vi "A_PID 15_MaxRR.vi"() -> ()   [LabVIEW 2011]
uses:
  <vilib>/DAQmx/read.llb/DAQmx Read (Analog 1D DBL 1Chan NSamp).vi
  <vilib>/DAQmx/write.llb/DAQmx Write (Analog DBL 1Chan 1Samp).vi
  <vilib>/DAQmx/create/channels.llb/DAQmx Create Channel (AI-Voltage-Basic).vi
  <vilib>/DAQmx/configure/timing.llb/DAQmx Timing (Sample Clock).vi
  <vilib>/DAQmx/create/channels.llb/DAQmx Create Channel (AO-Voltage-Basic).vi
  <vilib>/DAQmx/miscellaneous.llb/DAQmx Fill In Error Info.vi
  <vilib>/express/express arith-compare/Formula/XNode/ExpressFormulaBlockNode.xnode
  <vilib>/Analysis/NI_AALBase.lvlib
  Program Files (x86)/National Instruments/LabVIEW 2011/resource/objmgr/daqmx.rc
panel:
  in  "A2":dbl=97.0
  in  "A1":dbl=98.0
  in  "error in":cluster{"status":bool}
  in  "?":T1(tab)
  in  "Go":bool
  out "Time":dbl
  out "Thermistor Back":dbl
  out "Thermistor Block":dbl
  out "Vial Ramp rate":dbl format="%#_3g"
  in  "stop":bool
  out "XY Graph":cluster{"Y":dbl[], "Y":dbl[]}[](graph)
  out "Setpoint":dbl
  in  "Zero":dbl=-0.6
  in  "Pole":dbl=-10000000000000.0
  in  "PID Heating":T2={"proportional gain (Kc)"=27.0, "integral time (Ti, s)"=8.1, "derivative time (Td, s)"=0.0} {"derivative time (Td, s)" format="%.3f"; "integral time (Ti, s)" format="%.3f"; "proportional gain (Kc)" format="%.3f"}
  out "Set Pt RampRate":dbl
  out "Error":dbl
  in  "PID Cooling":T2={"proportional gain (Kc)"=33.0, "integral time (Ti, s)"=7.0, "derivative time (Td, s)"=0.0} {"derivative time (Td, s)" format="%.3f"; "integral time (Ti, s)" format="%.3f"; "proportional gain (Kc)" format="%.3f"}
  out "Controller output":cluster{"Time Out":dbl[], dbl[]}(graph)
  out "Power Circuit":cluster{"Time Out":dbl[], dbl[]}(graph)
  out "Voltage":dbl
  out "Ave RR Up":dbl
  out "Ave RR Down":dbl
  in  "Voltage Manual":dbl=5.0
  out "volt":dbl
  in  "A3":dbl=52.0
  in  "A4":dbl=55.0
  in  "T1":dbl=16.0
  in  "T2":dbl=2.0
  in  "T3":dbl=6.0
  in  "T4":dbl=6.0
  in  "T5":dbl=12.0
  in  "T6":dbl=6.0
  in  "T7":dbl=6.0
  in  "T8":dbl=6.0
  in  "T10":dbl=6.0
  in  "T9":dbl=6.0
  in  "A6":dbl=55.0
  in  "A5":dbl=52.0
  in  "Graph Range":dbl=150.0
  out "Rate":dbl
  in  "Period(ms)":dbl=20.0
  out "time":dbl
  # "PID"
  # "Lead-Lag Compensator"
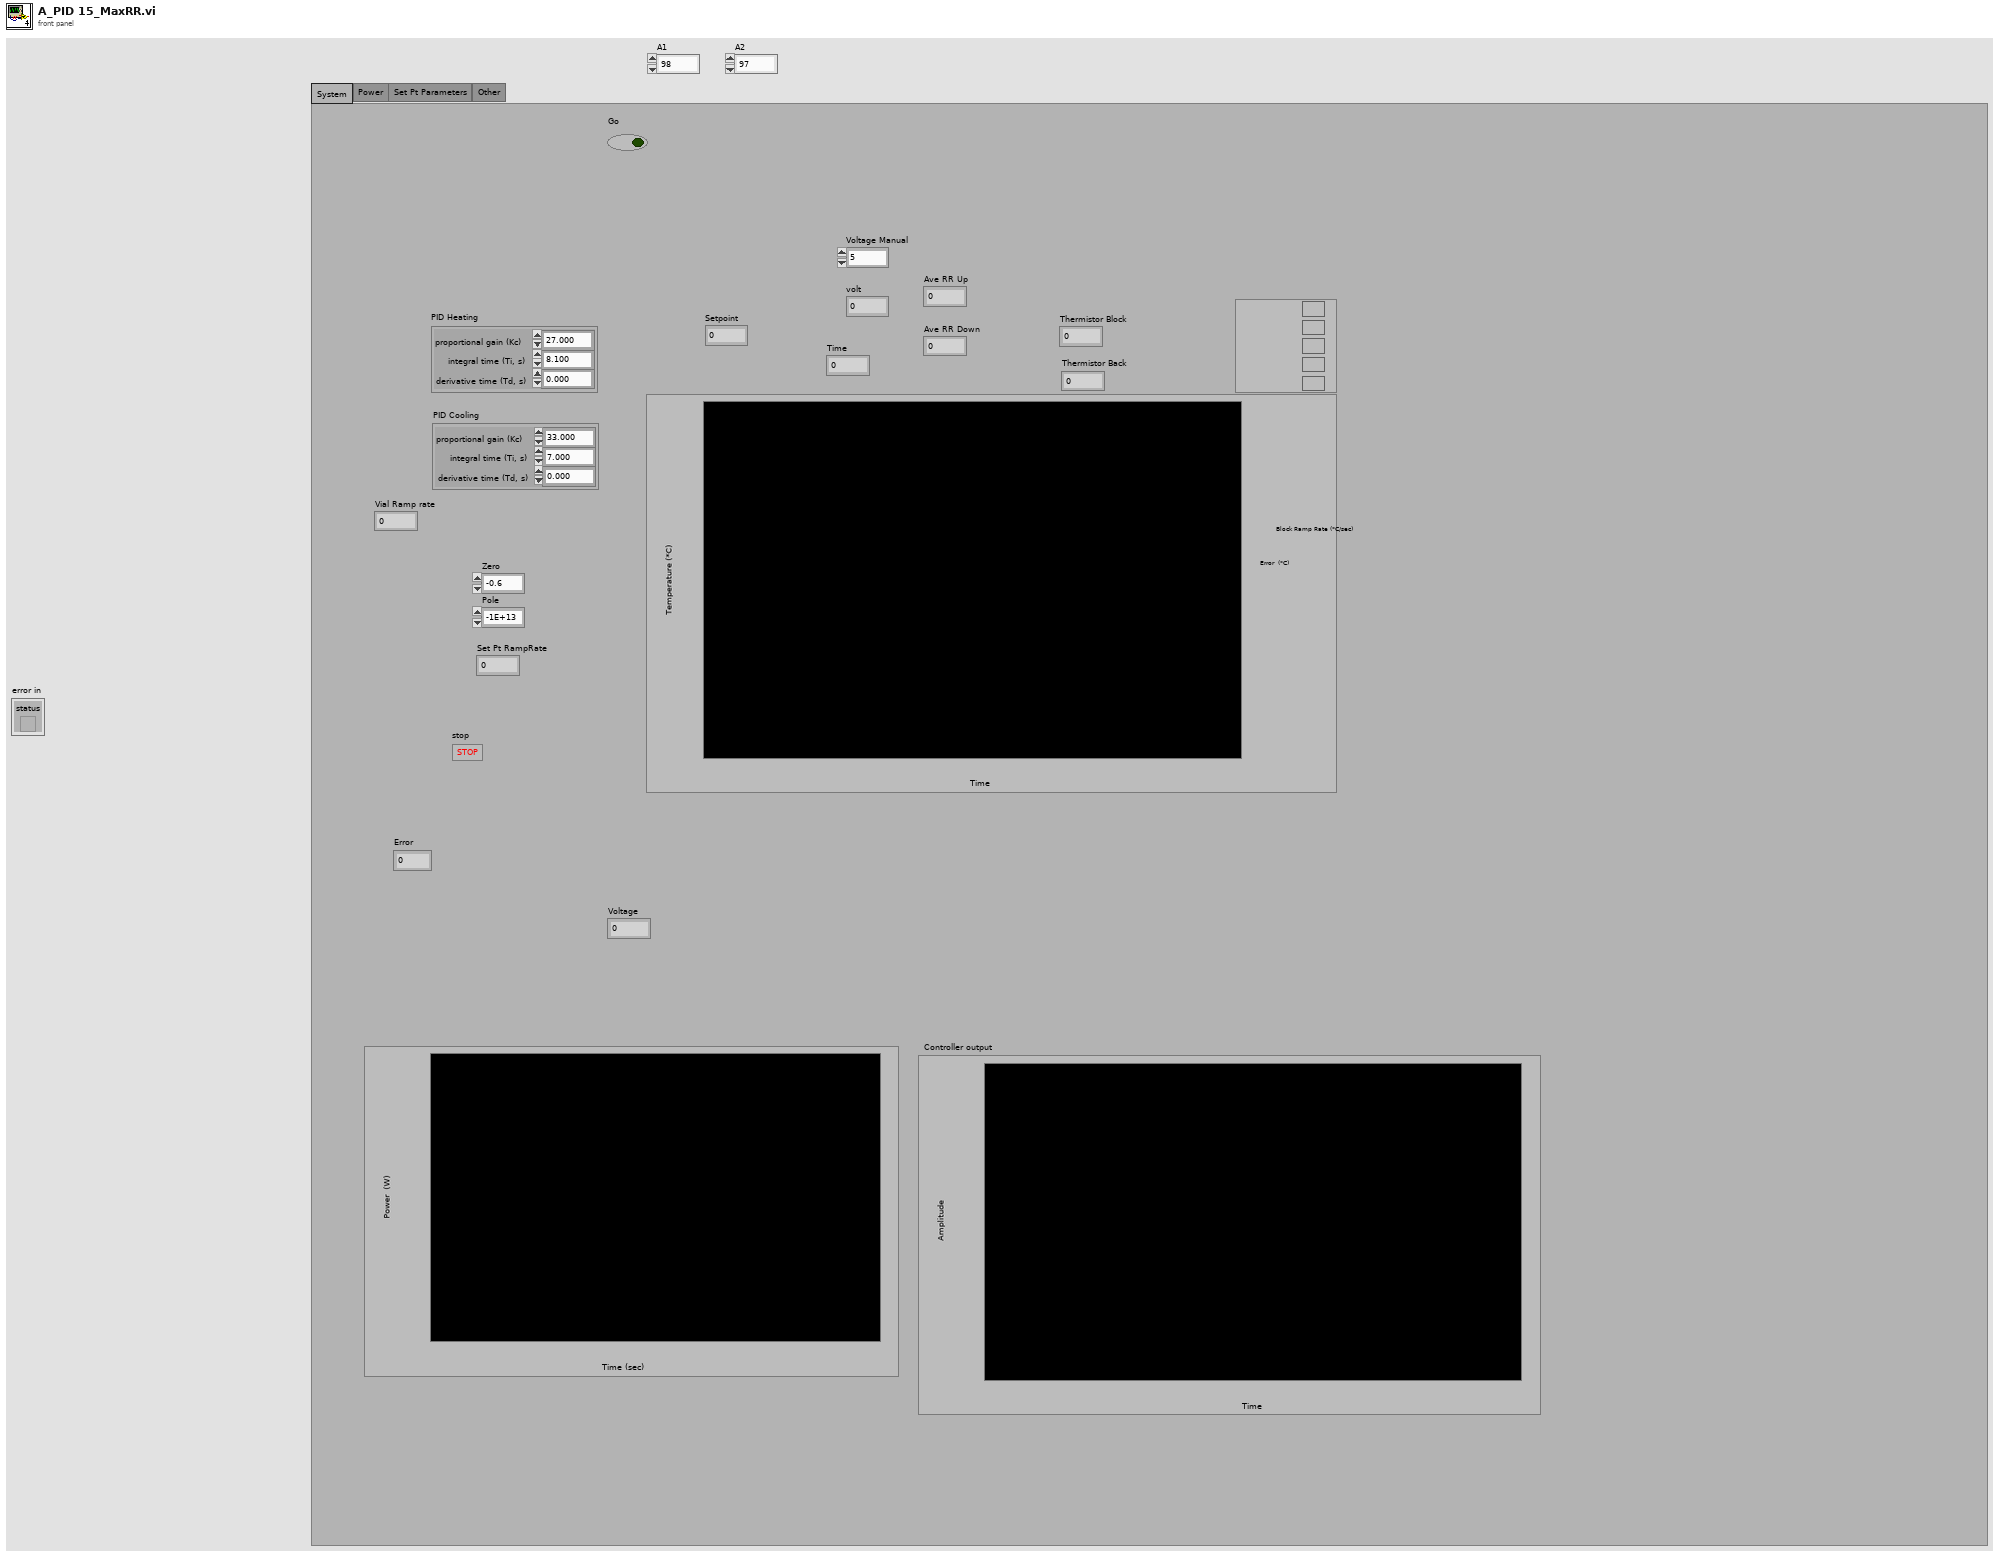
[diagram p1: front panel]
types:
  T1 = enum32{"System", "Power", "Set Pt Parameters", "Other"}
  T2 = cluster{"proportional gain (Kc)":dbl, "integral time (Ti, s)":dbl, "derivative time (Td, s)":dbl}
  T3 = enum16{"open", "replace", "create", "open or create", "replace or create", "replace or create with confirmation"}
  T4 = cluster{"x":dbl, "T1":dbl, "T2":dbl, "T3":dbl, "T4":dbl, "Te1":dbl, "Te2":dbl, "Te3":dbl, "Te4":dbl}
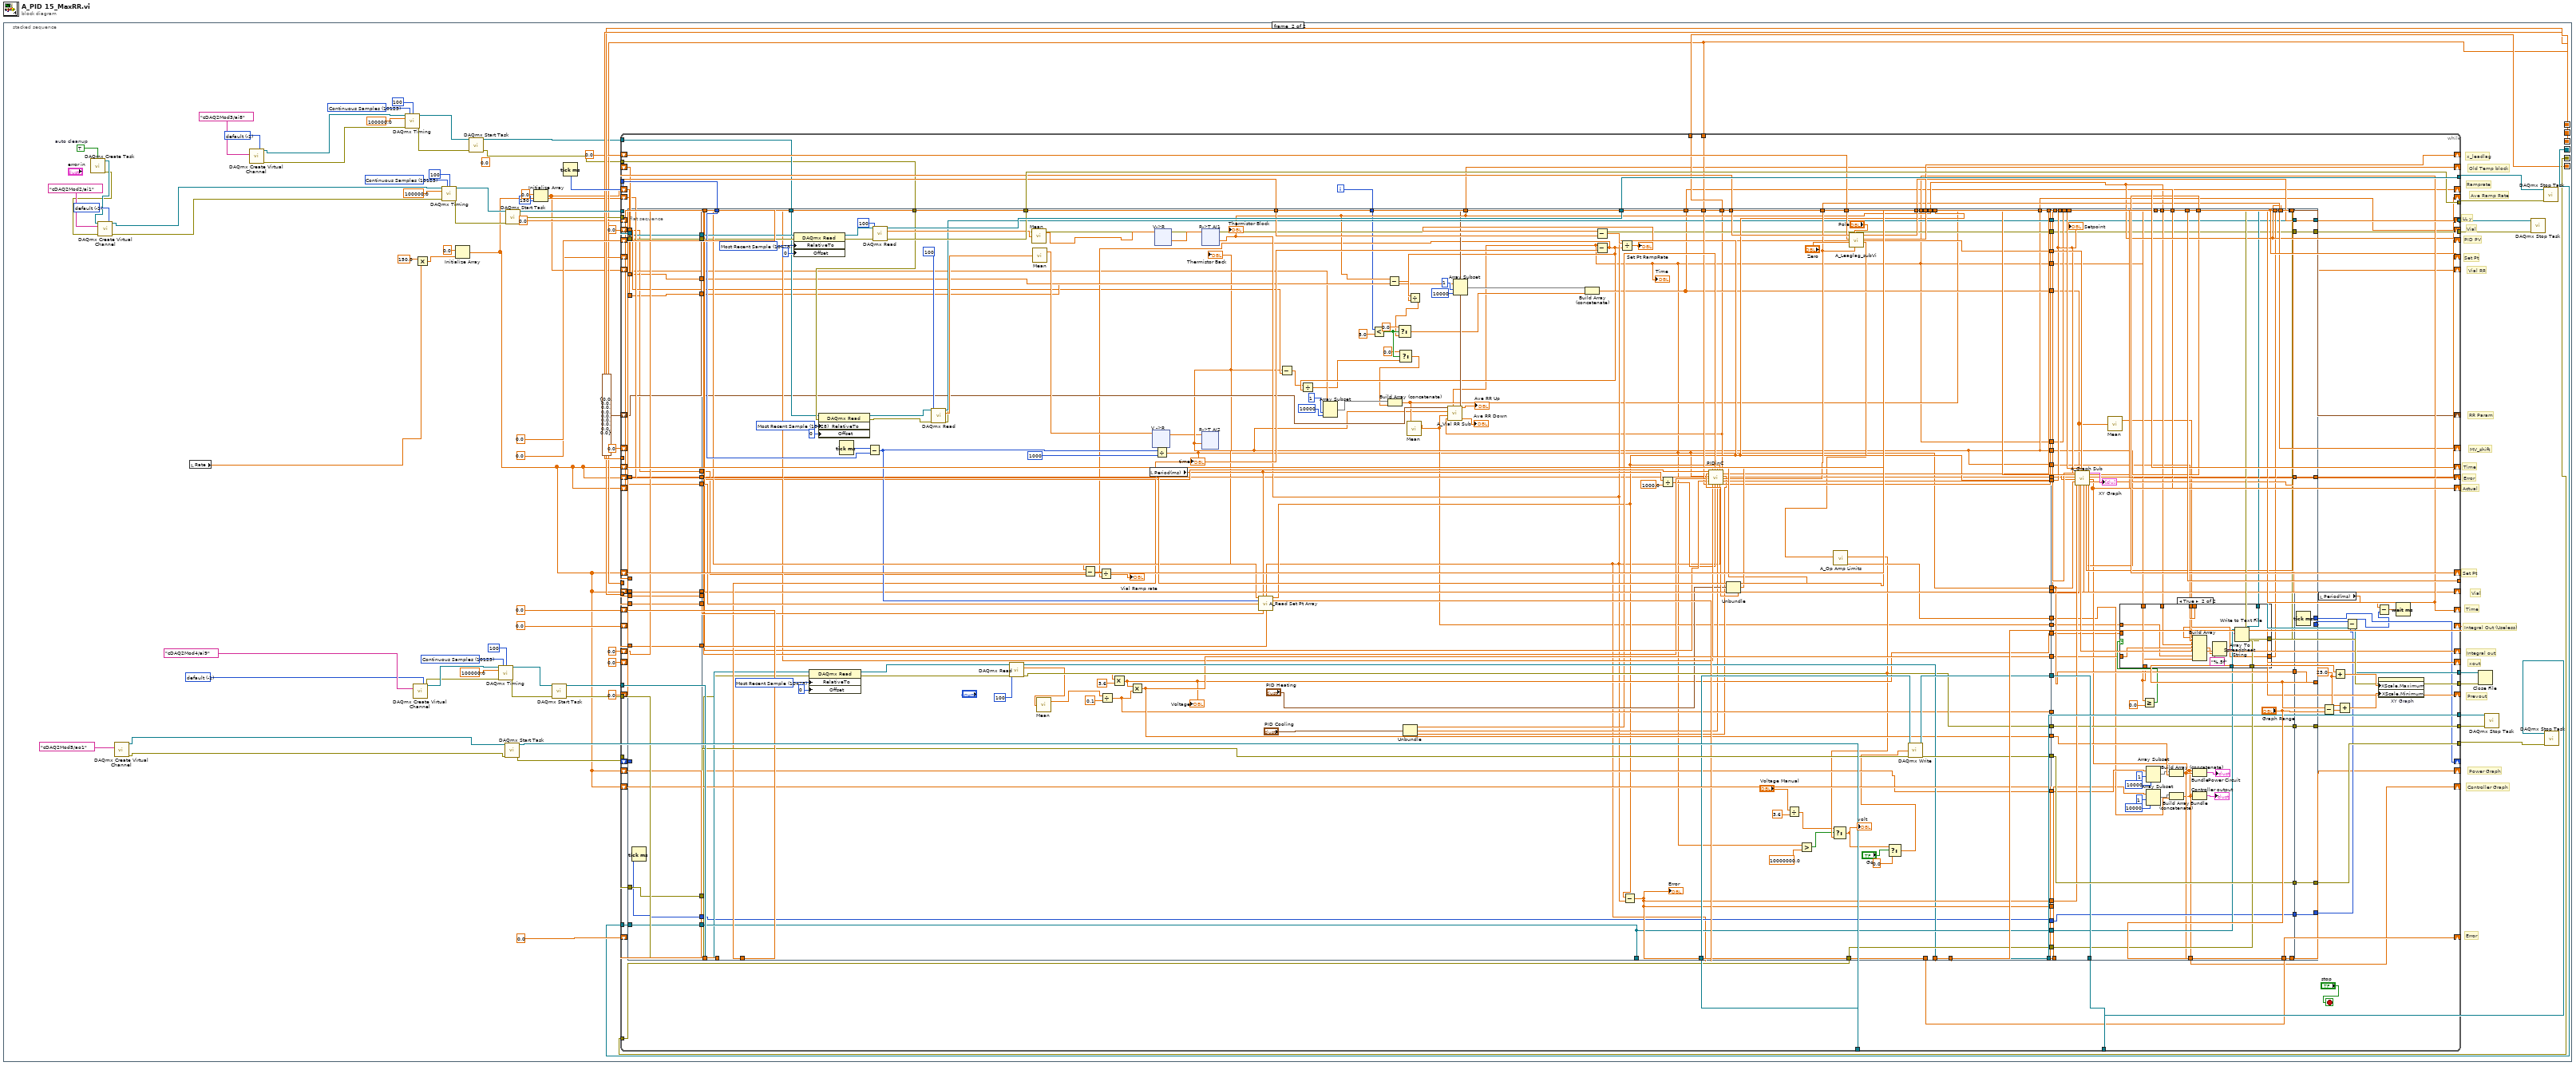
[diagram p0: block diagram]
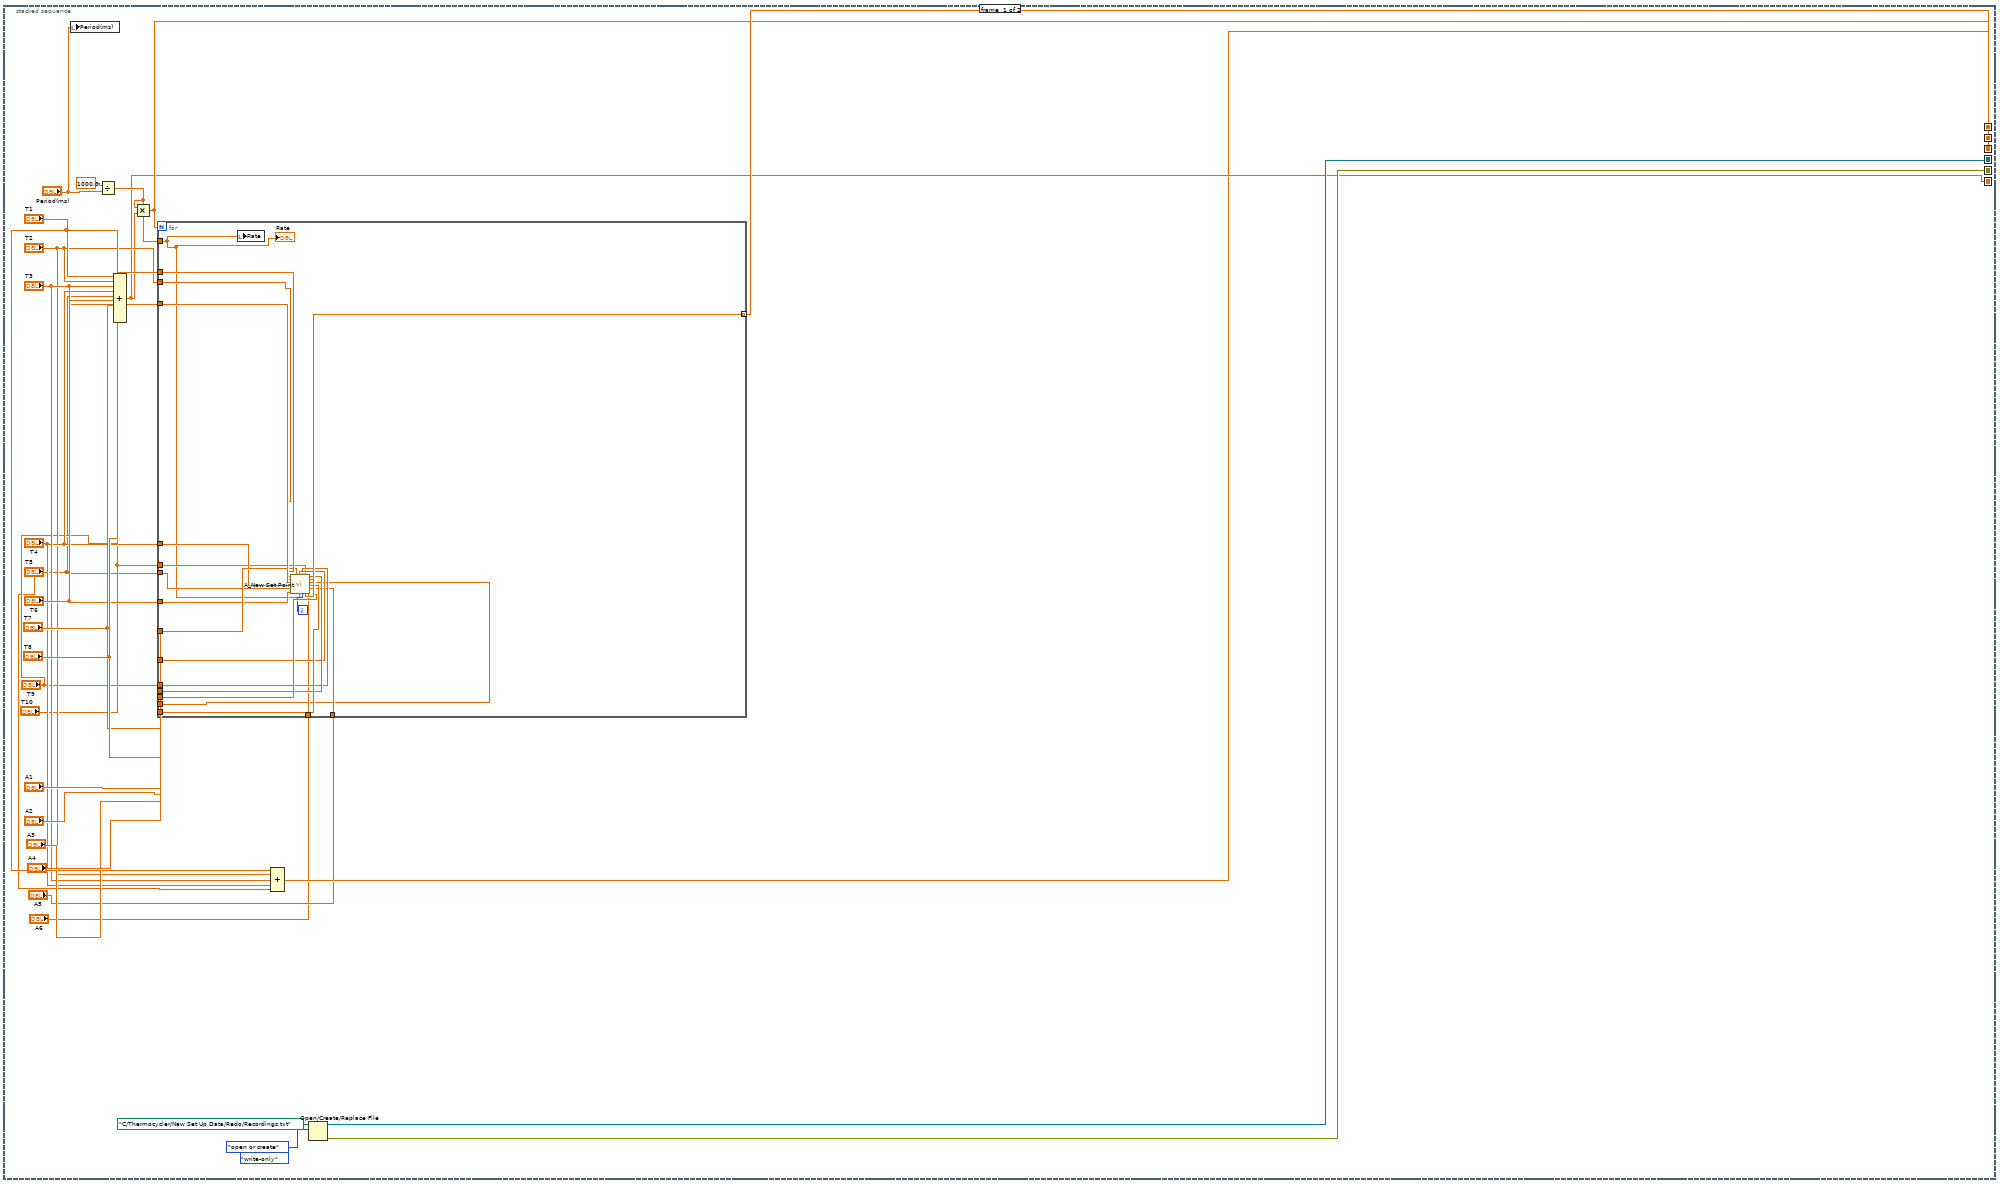
[diagram p2: hidden frame]
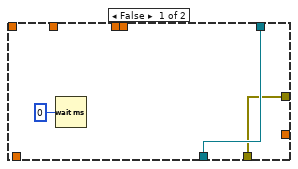
[diagram p3: hidden frame]
diagram:
  n1 = stacked-sequence {
    seq-local: [w19 _] -> [_ w113]
    seq-local: [w13 _] -> [_ w111]
    seq-local: [w6 _] -> [_ w67]
    seq-local: [w10 _] -> [_ w101]
    seq-local: [w9 _] -> [_ w100]
    seq-local: [w7 _] -> [_ w68]
    frame #0 {
      (unwired) enum16{"read/write", "read-only", "write-only"}."write-only" ("access (0:read/write)")
      n2 = local write "Period(ms)"("Period(ms)") -> ()
      n3 = Divide(x=1000.0, y="Period(ms)") -> (x/y=w14:dbl)
      n4 = Compound Arithmetic op=ADD("T1", "T2", "T3", "T4", "T5", "T6", "T7", "T8", "T9", "T10") -> (w7:dbl)
      n5 = Multiply(x=w14, y=w7) -> (x*y=w13:dbl)
      n6 = for {
        N: w13 -> [_]
        tunnel: "T1" -> [w44]
        tunnel: w14 -> [w28]
        tunnel: "T2" -> [w45]
        tunnel: "T3" -> [w46]
        tunnel: "T4" -> [w38]
        tunnel: "T5" -> [w39]
        tunnel: "T6" -> [w40]
        tunnel: "T7" -> [w41]
        tunnel: "T8" -> [w35]
        tunnel: [w43] -> w19 mode=indexing
        tunnel: "A1" -> [w36]
        tunnel: "A2" -> [w37]
        tunnel: "A3" -> [w30]
        tunnel: "A4" -> [w42]
        tunnel: "T9" -> [w34]
        tunnel: "T10" -> [w33]
        tunnel: "A5" -> [w32]
        tunnel: "A6" -> [w31]
        i -> [w29]
        n7 = local write "Rate"(w28) -> ()
        n8 = call "A_New Set Point.vi"("T1"=w44, "T2"=w45, "T3"=w46, "T4"=w38, "T5"=w39, "T6"=w40, "T7"=w41, "T8"=w35, "Period"=w28, "T9"=w34, "i"=w29, "T10"=w33, "A1"=w36, "A2"=w37, "A3"=w30, "A4"=w42, "A5"=w32, "A6"=w31) -> ("y"=w43:dbl)  [unwired: 1 in]
        "Rate" <- w28
      }
      n9 = Compound Arithmetic op=ADD("T1", "T2", "T3", "T4", "T5") -> (w6:dbl)
      n10 = Open/Create/Replace File(file path (use dialog)=path "C:/Thermocycler/New Set Up Data/Redo/Recordings.txt", operation (0:open)=T3."open or create") -> (refnum out=w10:refnum<file>, error out=w9:errorcluster)  [unwired: 2 in, 3 out]
    }
    frame #1 {
      w61 = -1 items=["default"=-1, "RSE"=10083, "NRSE"=10078, "Differential"=10106, "Pseudodifferential"=12529] ("input terminal configuration")
      (unwired) 0.0 ("y")
      w64 = 10123 items=["Finite Samples"=10178, "Continuous Samples"=10123, "Hardware Timed Single Point"=12522] ("sample mode")
      w84 = TRUE  # auto cleanup
      w86 = -1 items=["default"=-1, "RSE"=10083, "NRSE"=10078, "Differential"=10106, "Pseudodifferential"=12529] ("input terminal configuration")
      w93 = 10123 items=["Finite Samples"=10178, "Continuous Samples"=10123, "Hardware Timed Single Point"=12522] ("sample mode")
      w96 = -1 items=["default"=-1, "RSE"=10083, "NRSE"=10078, "Differential"=10106, "Pseudodifferential"=12529] ("input terminal configuration")
      w122 = 10123 items=["Finite Samples"=10178, "Continuous Samples"=10123, "Hardware Timed Single Point"=12522] ("sample mode")
      # "Vial RR"
      # "Vial"
      # "RR Param"
      # "Ave Ramp Rate"
      # "Ramprate"
      # "Old Temp block"
      # "Controller Graph"
      # "Power Graph"
      # "MV_shift"
      # "Prevout"
      # "xout"
      # "Integral out"
      # "Vial"
      # "Time"
      # "Integral Out (Useless)"
      # "Error"
      # "PID PV"
      # "Set Pt"
      # "x_leadlag"
      # "Set Pt"
      # "Actual"
      # "Error"
      # "Time"
      # "LL y"
      n11 = call <vilib>:"DAQmx Create Task.vi"("auto cleanup"=w84) -> ("task out"=w83:refnum<k21>, "error out"=w82:errorcluster)  [unwired: 13 in]
      n12 = call-poly <vilib>:"DAQmx Create Virtual Channel.vi"("task in"=w83, "input terminal configuration"=w86, "physical channels"=tag "cDAQ2Mod2/ai1", "error in"=w82) -> ("task out"=w66:refnum<k21>, "error out"=w65:errorcluster)  [unwired: 10 in]
      n13 = call-poly <vilib>:"DAQmx Create Virtual Channel.vi"("physical channels"=tag "cDAQ2Mod5/ao1") -> ("task out"=w76:refnum<k21>, "error out"=w75:errorcluster)  [unwired: 13 in]
      n14 = local read "Rate"() -> (w106:dbl)
      n15 = call-poly <vilib>:"DAQmx Create Virtual Channel.vi"("input terminal configuration"=w61, "physical channels"=tag "cDAQ2Mod3/ai8") -> ("task out"=w57:refnum<k21>, "error out"=w56:errorcluster)  [unwired: 12 in]
      n16 = call-poly <vilib>:"DAQmx Timing.vi"("task/channels in"=w57, "sample mode"=w64, "samples per channel"=100, "rate"=100000.0, "error in"=w56) -> ("task out"=w59:refnum<k21>, "error out"=w58:errorcluster)  [unwired: 9 in]
      n17 = call-poly <vilib>:"DAQmx Create Virtual Channel.vi"("input terminal configuration"=w96, "physical channels"=tag "cDAQ2Mod4/ai9") -> ("task out"=w95:refnum<k21>, "error out"=w94:errorcluster)  [unwired: 12 in]
      n18 = Multiply(x=150.0, y=w106) -> (x*y=w105:dbl)
      n19 = call-poly <vilib>:"DAQmx Timing.vi"("task/channels in"=w66, "sample mode"=w122, "samples per channel"=100, "rate"=100000.0, "error in"=w65) -> ("task out"=w80:refnum<k21>, "error out"=w79:errorcluster)  [unwired: 9 in]
      n20 = Initialize Array(0.0 ("element"), w105) -> (w49:dbl[])
      n21 = call <vilib>:"DAQmx Start Task.vi"("task/channels in"=w59, "error in"=w58) -> ("task out"=w55:refnum<k21>, "error out"=w54:errorcluster)  [unwired: 12 in]
      n22 = call-poly <vilib>:"DAQmx Timing.vi"("task/channels in"=w95, "sample mode"=w93, "samples per channel"=100, "rate"=100000.0, "error in"=w94) -> ("task out"=w78:refnum<k21>, "error out"=w77:errorcluster)  [unwired: 9 in]
      n23 = call <vilib>:"DAQmx Start Task.vi"("task/channels in"=w76, "error in"=w75) -> ("task out"=w112:refnum<k21>, "error out"=w118:errorcluster)  [unwired: 12 in]
      n24 = call <vilib>:"DAQmx Start Task.vi"("task/channels in"=w80, "error in"=w79) -> ("task out"=w120:refnum<k21>, "error out"=w81:errorcluster)  [unwired: 12 in]
      n25 = Initialize Array(0.0 ("element"), 150 ("dimension size")) -> (w48:dbl[])
      n26 = call <vilib>:"DAQmx Start Task.vi"("task/channels in"=w78, "error in"=w77) -> ("task out"=w90:refnum<k21>, "error out"=w89:errorcluster)  [unwired: 12 in]
      n27 = Tick Count (ms)() -> (millisecond timer value=w125:u32)
      n28 = while {
        tunnel: w125 -> [w263]
        shift-right: [w174] -> _
        shift-left: 0.0 ("data") -> [w241]
        shift-right: [w206] -> _
        shift-left: 0.0 -> [w260]
        tunnel: w81 -> [w258]
        tunnel: w120 -> [w257]
        tunnel: w118 -> [w254]
        tunnel: [w252] -> w117
        tunnel: [w249] -> w116
        tunnel: [w248] -> w115
        tunnel: [w247] -> w114
        tunnel: w113 -> [w246]
        tunnel: w112 -> [w244]
        tunnel: w111 -> [w242]
        shift-right: [w205] -> _
        shift-left: 0.0 ("Setpoint") -> [w214]
        shift-right: [w229] -> _
        shift-left: 0.0 ("Integral") -> [w238]
        tunnel: [w237] -> _
        shift-right: [w236] -> _
        shift-left: 0.0 -> [w235]
        shift-right: [w207] -> _
        shift-left: 0.0 ("y") -> [w233]
        tunnel: w67 -> [w231]
        shift-right: [w211] -> _
        shift-left: w49 -> [w227]
        shift-right: [w210] -> _
        shift-left: w49 -> [w224]
        shift-right: [w208] -> _
        shift-left: w49 -> [w223]
        shift-right: [w209] -> _
        shift-left: w49 -> [w228]
        shift-right: [w217] -> _
        shift-left: 0.0 ("LL x out") -> [w216]
        tunnel: w101 -> [w204]
        tunnel: w100 -> [w201]
        tunnel: [w199] -> w99
        tunnel: [w198] -> w98
        tunnel: w90 -> [w197]
        tunnel: w89 -> [w196]
        tunnel: [w195] -> w88
        tunnel: [w194] -> w87
        shift-right: [w189] -> _
        shift-left: w49 -> [w188]
        shift-right: [w184] -> _
        shift-left: 0.0 ("Integral out") -> [w180]
        shift-right: [w183] -> _
        shift-left: 0.0 ("x out") -> [w179]
        shift-right: [w182] -> _
        shift-left: 0.0 ("prev out") -> [w181]
        shift-right: [w178] -> _
        shift-left: 0.0 ("MV") -> [w177]
        shift-right: [w176] -> _
        shift-left: 0.0 ("Result") -> [w131]
        shift-right: [w168] -> _
        shift-left: _ -> [w167]
        shift-right: [w161] -> _
        shift-left: w49 -> [w163]
        shift-right: [w159] -> _
        shift-left: w49 -> [w160]
        tunnel: w68 -> [w156]
        tunnel: w67 -> [w155]
        tunnel: w55 -> [w154]
        tunnel: w54 -> [w147]
        tunnel: [w151] -> w53
        tunnel: [w148] -> w52
        shift-right: [w146] -> _
        shift-left: _ -> [w145]
        shift-right: [w143] -> _
        shift-left: w48 -> [w142]
        shift-right: [w139] -> _
        shift-left: w49 -> [w137]
        shift-right: [w133] -> _
        shift-left: T4 {"x"=0.0, "T1"=0.0, "T2"=0.0, "T3"=0.0, "T4"=0.0, "Te1"=0.0, "Te2"=0.0, "Te3"=0.0, "Te4"=0.0} ("Param out") -> [w132]
        shift-right: [w130] -> _
        shift-left: w48 -> [w129]
        i -> [w127]
        stop <- "stop" stop-if-true
        w222 = 25.0 ("y")
        n29 = flat-sequence {
          tunnel: [w277] -> w259
          tunnel: w258 -> [w277]
          tunnel: w257 -> [w274]
          tunnel: [w274] -> w256
          tunnel: [w276] -> w255
          tunnel: w254 -> [w276]
          tunnel: w246 -> [w275]
          tunnel: [w275] -> w245
          tunnel: [w273] -> w243
          tunnel: w242 -> [w273]
          tunnel: [w272] -> w239
          tunnel: w238 -> [w272]
          tunnel: [w271] -> w232
          tunnel: w231 -> [w271]
          tunnel: w204 -> [w270]
          tunnel: [w270] -> w203
          tunnel: w188 -> [w269]
          tunnel: [w269] -> w187
          tunnel: [w268] -> w175
          tunnel: w131 -> [w268]
          tunnel: [w267] -> w172
          tunnel: w167 -> [_]
          tunnel: w145 -> [w266]
          tunnel: [w266] -> w144
          tunnel: w142 -> [w265]
          tunnel: [w265] -> w141
          tunnel: w137 -> [w264]
          tunnel: [w264] -> w136
          tunnel: w263 -> [w408]
          tunnel: [w340] -> w262
          tunnel: [w282] -> w261
          tunnel: [w282] -> w206
          tunnel: w260 -> [w385]
          tunnel: w259 -> [w380]
          tunnel: w256 -> [w406]
          tunnel: w255 -> [w405]
          tunnel: [w404] -> w253
          tunnel: [w403] -> w250
          tunnel: [w402] -> w248
          tunnel: [w401] -> w247
          tunnel: w245 -> [w400]
          tunnel: w244 -> [w399]
          tunnel: w243 -> [w398]
          tunnel: [w323] -> w174
          tunnel: w241 -> [w397]
          tunnel: [w323] -> w240
          tunnel: w214 -> [w389]
          tunnel: [w340] -> w205
          tunnel: [w396] -> w229
          tunnel: w239 -> [w395]
          tunnel: [w323] -> _
          tunnel: [w388] -> w236
          tunnel: w235 -> [_]
          tunnel: [w388] -> w234
          tunnel: [w391] -> w207
          tunnel: w233 -> [w392]
          tunnel: [w386] -> w217
          tunnel: w232 -> [_]
          tunnel: [w282] -> w226
          tunnel: [w388] -> w225
          tunnel: w216 -> [w387]
          tunnel: w203 -> [w384]
          tunnel: [w384] -> _
          tunnel: [w384] -> w202
          tunnel: w201 -> [w383]
          tunnel: [w383] -> w200
          tunnel: w197 -> [w382]
          tunnel: w196 -> [w379]
          tunnel: [w375] -> w195
          tunnel: [w374] -> w193
          tunnel: [w371] -> w191
          tunnel: [w371] -> w190
          tunnel: w187 -> [w370]
          tunnel: [w370] -> w186
          tunnel: [w300] -> w185
          tunnel: [w364] -> w184
          tunnel: [w363] -> w183
          tunnel: [w362] -> w182
          tunnel: w181 -> [w361]
          tunnel: w180 -> [w360]
          tunnel: w179 -> [w359]
          tunnel: [w358] -> w178
          tunnel: w177 -> [w357]
          tunnel: [w300] -> w176
          tunnel: w175 -> [w356]
          tunnel: [w300] -> w173
          tunnel: w172 -> [w351]
          tunnel: [w351] -> w171
          tunnel: w163 -> [w350]
          tunnel: [w350] -> w162
          tunnel: [w348] -> w158
          tunnel: [w347] -> w157
          tunnel: w156 -> [w308]
          tunnel: w155 -> [w342]
          tunnel: w154 -> [w327]
          tunnel: [w332] -> w153
          tunnel: [w331] -> w150
          tunnel: w147 -> [w328]
          tunnel: [w323] -> w146
          tunnel: w144 -> [w322]
          tunnel: [w318] -> w143
          tunnel: w141 -> [w319]
          tunnel: [w318] -> w140
          tunnel: w136 -> [w317]
          tunnel: [w317] -> w135
          tunnel: [w314] -> w134
          tunnel: [w311] -> w133
          tunnel: w132 -> [w310]
          tunnel: w131 -> [w306]
          tunnel: [w302] -> w130
          tunnel: w129 -> [w301]
          tunnel: [w287] -> w128
          tunnel: w127 -> [w293]
          tunnel: [w282] -> w126
          tunnel: w262 -> [w490]
          tunnel: w261 -> [w480]
          tunnel: w253 -> [w503]
          tunnel: [w503] -> w251
          tunnel: w250 -> [w502]
          tunnel: [w502] -> w249
          tunnel: w240 -> [w492]
          tunnel: [w480] -> _
          tunnel: [w490] -> w237
          tunnel: w234 -> [_]
          tunnel: "Graph Range" -> [_]
          tunnel: [w500] -> w209
          tunnel: w228 -> [w499]
          tunnel: w227 -> [w498]
          tunnel: [w462] -> w211
          tunnel: w226 -> [w491]
          tunnel: w225 -> [w497]
          tunnel: w224 -> [w496]
          tunnel: [w495] -> w210
          tunnel: [w494] -> w208
          tunnel: w223 -> [w493]
          tunnel: [w491] -> w221
          tunnel: w206 -> [w487]
          tunnel: w205 -> [w486]
          tunnel: w174 -> [_]
          tunnel: w202 -> [w485]
          tunnel: w200 -> [w484]
          tunnel: [w483] -> w199
          tunnel: [w482] -> w198
          tunnel: w193 -> [w481]
          tunnel: [w481] -> w192
          tunnel: w191 -> [w467]
          tunnel: w190 -> [w479]
          tunnel: [w478] -> w189
          tunnel: w186 -> [w477]
          tunnel: w185 -> [w476]
          tunnel: w174 -> [w475]
          tunnel: w173 -> [w473]
          tunnel: w171 -> [w474]
          tunnel: [w474] -> w170
          tunnel: w162 -> [w466]
          tunnel: [w465] -> w161
          tunnel: w160 -> [w459]
          tunnel: [w458] -> w159
          tunnel: w158 -> [w457]
          tunnel: w157 -> [_]
          tunnel: w153 -> [w456]
          tunnel: [w456] -> w152
          tunnel: w150 -> [w455]
          tunnel: [w455] -> w149
          tunnel: w140 -> [w452]
          tunnel: [w454] -> w138
          tunnel: w135 -> [w453]
          tunnel: w134 -> [w461]
          tunnel: w128 -> [w450]
          tunnel: w126 -> [w449]
          tunnel: [w524] -> w213
          tunnel: [w528] -> w252
          tunnel: w251 -> [w528]
          tunnel: w221 -> [w527]
          tunnel: [w527] -> w219
          tunnel: [w526] -> w194
          tunnel: w192 -> [w526]
          tunnel: w170 -> [w525]
          tunnel: [w525] -> w169
          tunnel: [w524] -> w168
          tunnel: w152 -> [w523]
          tunnel: [w523] -> w151
          tunnel: w149 -> [w522]
          tunnel: [w522] -> w148
          tunnel: [w521] -> w139
          tunnel: w138 -> [w521]
          frame #0 {
            n30 = Tick Count (ms)() -> (millisecond timer value=w267:u32)
          }
          frame #1 {
            w329 = 10428 items=["First Sample"=10424, "Current Read Position"=10425, "Reference Trigger"=10426, "First Pretrigger Sample"=10427, "Most Recent Sample"=10428] ("RelativeTo")
            w376 = 10428 items=["First Sample"=10424, "Current Read Position"=10425, "Reference Trigger"=10426, "First Pretrigger Sample"=10427, "Most Recent Sample"=10428] ("RelativeTo")
            w413 = 10428 items=["First Sample"=10424, "Current Read Position"=10425, "Reference Trigger"=10426, "First Pretrigger Sample"=10427, "Most Recent Sample"=10428] ("RelativeTo")
            n31 = property class="DAQmx Read"(reference=w406, error in=w380, "RelativeTo"=w413, "Offset"=0) -> (reference out=w411:refnum<k21>, error out=w410:errorcluster)
            n32 = property class="DAQmx Read"(reference=w382, error in=w379, "RelativeTo"=w376, "Offset"=0) -> (reference out=w381:refnum<k21>, error out=w378:errorcluster)
            n33 = property class="DAQmx Read"(reference=w327, error in=w328, "RelativeTo"=w329, "Offset"=0) -> (reference out=w326:refnum<k21>, error out=w325:errorcluster)
            n34 = Tick Count (ms)() -> (millisecond timer value=w414:u32)
            n35 = Subtract(x=w414, y=w408) -> (x-y=w390:u32)
            n36 = call-poly <vilib>:"DAQmx Read.vi"("task/channels in"=w411, "number of samples per channel"=100, "error in"=w410) -> ("task out"=w402:refnum<k21>, "data"=w335:dbl[], "error out"=w401:errorcluster)  [unwired: 10 in]
            n37 = call-poly <vilib>:"DAQmx Read.vi"("task/channels in"=w326, "number of samples per channel"=100, "error in"=w325) -> ("task out"=w332:refnum<k21>, "data"=w333:dbl[], "error out"=w331:errorcluster)  [unwired: 10 in]
            n38 = call-poly <vilib>:"DAQmx Read.vi"("task/channels in"=w381, "number of samples per channel"=100, "error in"=w378) -> ("task out"=w375:refnum<k21>, "data"=w337:dbl[], "error out"=w374:errorcluster)  [unwired: 10 in]
            n39 = call <vilib>:"Mean.vi"("X"=w335) -> ("mean"=w339:dbl)  [unwired: 1 out]
            n40 = call <vilib>:"Mean.vi"("X"=w333) -> ("mean"=w369:dbl)  [unwired: 1 out]
            n41 = call <vilib>:"Mean.vi"("X"=w337) -> ("mean"=w336:dbl)  [unwired: 1 out]
            n42 = Divide(x=w336, y=0.1) -> (x/y=w347:dbl)
            n43 = local read "Period(ms)"() -> (w354:dbl)
            n44 = xnode "V ->R"("V"=w369) -> ("Result"=w299:dbl)  [unwired: 1 in, 1 out]
            n45 = xnode "V->R"("V"=w339) -> ("Result"=w416:dbl)  [unwired: 1 in, 1 out]
            n46 = Divide(x=w390, y=1000) -> (x/y=w282:dbl)
            "time" <- w282
            "Time" <- w282
            n47 = xnode "R->T AI2"("R"=w299) -> ("Result"=w300:dbl)  [unwired: 1 in, 1 out]
            "Thermistor Back" <- w300
            n48 = Subtract(x=w300, y=w356) -> (x-y=w355:dbl)
            n49 = xnode "R->T AI1"("R"=w416) -> ("Result"=w323:dbl)  [unwired: 1 in, 1 out]
            "Thermistor Block" <- w323
            n50 = call "A_Read Set Pt Array.vi"("Previous y"=w397, "Period(ms)"=w354, "Result"=w323, "dt"=w390, "y array"=w400, "arraysize"=w398, "Integral in"=w395) -> ("Set Pt Out"=w340:dbl, "Integral out"=w396:dbl)  [unwired: 7 in]
            n51 = Subtract(x=w300, y=w306) -> (x-y=w305:dbl)
            n52 = Array Subset(array=w301, index=1, length=10000) -> (w307:dbl[])
            n53 = Less?(x=w293, y=5.0) -> (x < y?=w291:bool)
            n54 = Subtract(x=w323, y=w322) -> (x-y=w324:dbl)
            n55 = Unbundle("PID Cooling") -> ("proportional gain (Kc)"=w345:dbl, "integral time (Ti, s)"=w343:dbl, "derivative time (Td, s)"=w344:dbl)
            n56 = Array Subset(array=w319, index=1, length=10000) -> (w320:dbl[])
            n57 = Subtract(x=w340, y=w389) -> (x-y=w407:dbl)
            n58 = Subtract(x=w282, y=w385) -> (x-y=w309:dbl)
            n59 = Divide(x=w355, y=w309) -> (x/y=→"Vial Ramp rate":dbl)
            n60 = Divide(x=w305, y=w309) -> (x/y=w286:dbl)
            n61 = Select(t=0.0, s=w291, f=w286) -> (s? t:f=w285:dbl)
            n62 = Build Array (concatenate)(w307, w285) -> (w302:dbl[])
            n63 = call <vilib>:"Mean.vi"("X"=w302) -> ("mean"=w287:dbl)  [unwired: 1 out]
            n64 = Divide(x=w324, y=w309) -> (x/y=w289:dbl)
            n65 = Select(t=0.0, s=w291, f=w289) -> (s? t:f=w288:dbl)
            n66 = call "A_Vial RR Sub.vi"("t"=w282, "TotalTime"=w308, "Vial Slope"=w287, "Vial Temp"=w300, "Param in"=w310) -> ("Ave RR Down"=→"Ave RR Down":dbl, "Param out"=w311:T4, "Ave RR Up"=→"Ave RR Up":dbl)  [unwired: 4 in]
            n67 = Build Array (concatenate)(w320, w288) -> (w318:dbl[])
            n68 = Divide(x=w407, y=w309) -> (x/y=→"Set Pt RampRate":dbl)
            n69 = Subtract(x=w340, y=w323) -> (x-y=w388:dbl)
            "Error" <- w388
            n70 = Divide(x=w354, y=1000.0) -> (x/y=w353:dbl)
            n71 = Unbundle("PID Heating") -> ("proportional gain (Kc)"=w366:dbl, "integral time (Ti, s)"=w367:dbl, "derivative time (Td, s)"=w368:dbl)
            n72 = call "PIDinC.vi"("MV in"=w357, "D"=w368, "Time"=w282, "Integral in"=w360, "prev in"=w361, "Rising half"=w342, "I"=w367, "x in"=w359, "P2"=w345, "dt"=w353, "P"=w366, "I2"=w343, "Set Point"=w340, "PV"=w323, "Total Time"=w308, "D2"=w344) -> ("Integral out"=w364:dbl, "MV"=w358:dbl, "prev out"=w362:dbl, "x out"=w363:dbl)
            n73 = Divide(x="Voltage Manual", y=3.6) -> (x/y=w295:dbl)
            n74 = Greater?(x=w282, y=10000000.0) -> (0:w283:bool)
            n75 = call "A_Leaglag_subVi.vi"("LL x"=w358, "Pole"="Pole", "Zero"="Zero", "LL x_prev"=w387, "LL y_prev"=w392) -> ("y*inv_gain"=w315:dbl, "LL x out"=w386:dbl, "LL y"=w391:dbl)  [unwired: 4 in]
            n76 = call "A_Op Amp Limits.vi"("Lead Lag"=w315) -> ("Controller Output"=w314:dbl, "Write DAQmx"=w298:dbl)  [unwired: 9 in]
            n77 = Multiply(x=w298, y=3.6) -> (x*y=w348:dbl)
            "Voltage" <- w348
            n78 = Multiply(x=w348, y=w347) -> (x*y=w371:dbl)
            n79 = Select(t=w295, s=w283, f=w298) -> (s? t:f=w280:dbl)
            "volt" <- w280
            n80 = Select(t=w280, s="Go", f=0.0) -> (s? t:f=w278:dbl)
            n81 = call-poly <vilib>:"DAQmx Write.vi"("task/channels in"=w399, "data"=w278, "error in"=w405) -> ("task out"=w403:refnum<k21>, "error out"=w404:errorcluster)  [unwired: 10 in, 1 out]
          }
          frame #2 {
            n82 = call "A_Graph Sub.vi"("Set Point Shift"=w499, "New Set Pt"=w490, "Ramp Rate Shift"=w453, "Time Shift"=w498, "New Time"=w491, "New Error"=w497, "New Ramp Rate"=w452, "Error Shift"=w496, "New Actual"=w492, "Actual Shift"=w493, "New Vial"=w476, "Vial Shift"=w477) -> ("Vial Out"=w478:dbl[], "Actual Out"=w494:dbl[], "Graph Out"=→"XY Graph":cluster{dbl[], dbl[]}[], "Set Pt Out"=w500:dbl[], "Ramp Rate Out"=w454:dbl[], "Time Out"=w462:dbl[], "Error Out"=w495:dbl[])  [unwired: 1 in]
            n83 = call <vilib>:"Mean.vi"("X"=w452) -> ("mean"=w451:dbl)  [unwired: 1 out]
            n84 = Greater Or Equal?(x=w487, y=0.0) -> (x >= y?=w488:bool)
            n85 = case shown="True" w488 {
              tunnel: w487 -> [_ _]
              tunnel: w486 -> [_ w510]
              tunnel: w485 -> [w505 w520]
              tunnel: w484 -> [w504 w519]
              tunnel: [w504 w518] -> w483
              tunnel: [w505 w517] -> w482
              tunnel: w479 -> [_ w513]
              tunnel: w475 -> [_ w512]
              tunnel: w473 -> [_ w511]
              tunnel: w457 -> [_ _]
              tunnel: w451 -> [_ w509]
              tunnel: w450 -> [_ w508]
              tunnel: w449 -> [_ w507]
              frame False {
                n86 = Wait (ms)(milliseconds to wait=u32 0) -> ()  [unwired: 1 out]
              }
              frame True {
                n87 = Build Array(w510, w511, w512, w513, w509, w508, w507) -> (w516:dbl[])
                n88 = Array To Spreadsheet String(array=w516, 3:"%.5f" ("format string")) -> (spreadsheet string=w514:string)  [unwired: 1 out]
                n89 = Write to Text File(file (use dialog)=w520, text=w514, error in=w519) -> (refnum out=w517:refnum<file>, error out=w518:errorcluster)  [unwired: 1 in, 1 out]
              }
            }
            n90 = Array Subset(array=w459, index=1, length=10000) -> (w460:dbl[])
            n91 = Array Subset(array=w466, index=1, length=10000) -> (w464:dbl[])
            n92 = Build Array (concatenate)(w460, w461) -> (w458:dbl[])
            n93 = Build Array (concatenate)(w464, w467) -> (w465:dbl[])
            n94 = Bundle("Time Out"=w462, w458) -> (→"Controller output":cluster{"Time Out":dbl[], dbl[]})  [unwired: 1 in]
            n95 = Bundle("Time Out"=w462, w465) -> (→"Power Circuit":cluster{"Time Out":dbl[], dbl[]})  [unwired: 1 in]
            "Setpoint" <- w490
          }
          frame #3 {
            n96 = Tick Count (ms)() -> (millisecond timer value=w524:u32)
          }
        }
        n97 = local read "Period(ms)"() -> (w166:dbl)
        n98 = Subtract(x=w219, y="Graph Range") -> (x-y=w230:dbl)
        n99 = Add(x=w219, y=w222) -> (x+y=w220:dbl)
        n100 = Add(x=w222, y=w230) -> (x+y=w218:dbl)
        n101 = Subtract(x=w213, y=w169) -> (x-y=w164:u32)
        n102 = Subtract(x=w166, y=w164) -> (x-y=w165:dbl)
        n103 = property on="XY Graph" class="XYGraph (strict)"("XScale.Maximum"=w220, "XScale.Minimum"=w218) -> ()  [unwired: 2 in, 2 out]
        n104 = Wait (ms)(milliseconds to wait=w165) -> ()  [unwired: 1 out]
      }
      n105 = Close File(refnum=w98, error in=w99) -> ()  [unwired: 2 out]
      n106 = call <vilib>:"DAQmx Stop Task.vi"("task/channels in"=w88, "error in"=w87) -> ()  [unwired: 12 in, 2 out]
      n107 = call <vilib>:"DAQmx Stop Task.vi"("task/channels in"=w53, "error in"=w52) -> ()  [unwired: 12 in, 2 out]
      n108 = call <vilib>:"DAQmx Stop Task.vi"("task/channels in"=w115, "error in"=w114) -> ()  [unwired: 12 in, 2 out]
      n109 = call <vilib>:"DAQmx Stop Task.vi"("task/channels in"=w116, "error in"=w117) -> ()  [unwired: 12 in, 2 out]
    }
  }
